vi "DMA Odometry Calculate.vi"(10 "Reset?":bool, 11 "Encoder Factor":dbl=1.0) -> (2 "Data Lost?":bool, 3 "Pose":T1)   [LabVIEW 2019]
uses:
  <vilib>/Rock Robotics/WPI/ThirdParty/WPILib Extensions/Geometry/Typedef/Pose2d.ctl
  <vilib>/Rock Robotics/WPI/ThirdParty/WPILib Extensions/Geometry/Typedef/Translation2d.ctl
  <vilib>/Rock Robotics/WPI/ThirdParty/WPILib Extensions/Geometry/Typedef/Rotation2d.ctl
  1db27cf9-0598-4eea-a655-fd467044f8ee.vi
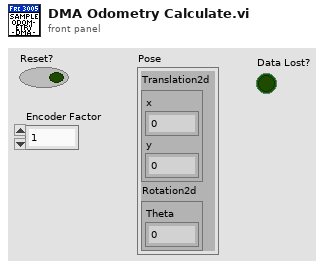
[diagram p1: front panel]
types:
  T1 = typedef "Pose2d.ctl" = cluster{"Translation2d":T2, "Rotation2d":T3}
  T2 = typedef "Translation2d.ctl" = cluster{"x":dbl, "y":dbl}
  T3 = typedef "Rotation2d.ctl" = cluster{"Theta":dbl}
  T4 = cluster{"Encoder R":i32, "Encoder L":i32, "Timestamp":u32}[]
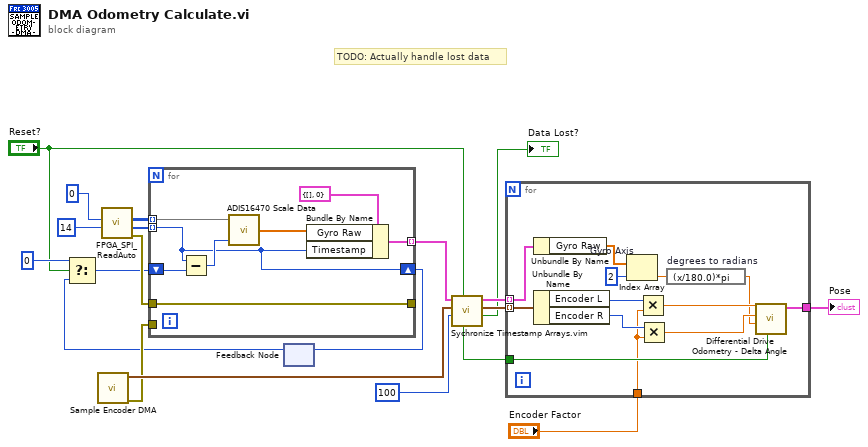
[diagram p0: block diagram]
diagram:
  # "TODO: Actually handle lost data"
  n1 = call "Sample Encoder DMA.vi"() -> ("error out"=w13:errorcluster, "Array"=w14:T4)  [unwired: 10 in]
  n2 = call <vilib>:"FPGA_SPI_ReadAuto.vi"("Bytes per Sample"=u32 14 ("Bytes Per Sample"), "Samples to Read"=u32 0) -> ("error out"=w12:errorcluster, "Timestamps"=w11:u32[], "Data"=w10:u8[][])  [unwired: 6 in, 1 out]
  n3 = feedback #1() -> (w4:u32)  [unwired: 1 in]
  n4 = Select(t=u32 0, s="Reset?", f=w4) -> (s? t:f=w3:u32)
  n5 = for {
    tunnel: w10 -> [w26] mode=indexing
    tunnel: w11 -> [w21] mode=indexing
    tunnel: w12 -> [w27]
    tunnel: [w27] -> _
    tunnel: w13 -> [_]
    tunnel: [w23] -> w15 mode=indexing
    shift-right: [w21] -> w5
    shift-left: w3 -> [w20]
    n6 = Subtract(x=w21, y=w20) -> (x-y=w22:u32)
    n7 = call "ADIS16470 Scale Data.vi"("TimeStamp"=w22, "Data In"=w26) -> ("Scaled Data Out"=w24:dbl[])  [unwired: 3 in]
    n8 = Bundle By Name(cluster=cluster{"Gyro Raw":dbl[], "Timestamp":u32} {"Gyro Raw"=[], "Timestamp"=0}, "Gyro Raw"=w24, "Timestamp"=w21) -> (w23:cluster{"Gyro Raw":dbl[], "Timestamp":u32})
  }
  n9 = feedback-in #1(w5) -> ()
  n10 = call "Sychronize Timestamp Arrays.vim"("Reset? (F)"="Reset?", "Timestamp Tolerance"=100, "Dataset 2"=w14, "Dataset 1"=w15) -> ("Data Lost?"=→"Data Lost?":bool, "Dataset 2 Out"=w17:T4, "Dataset 1 Out"=w16:cluster{"Gyro Raw":dbl[], "Timestamp":u32}[])  [unwired: 5 in]
  n11 = for {
    tunnel: w16 -> [w40] mode=indexing
    tunnel: w17 -> [w39] mode=indexing
    tunnel: "Reset?" -> [w35]
    tunnel: [w34] -> w18
    tunnel: "Encoder Factor" -> [w29]
    w37 = 2  # Gyro Axis
    n12 = Unbundle By Name(w40) -> ("Gyro Raw"=w38:dbl[])
    n13 = Unbundle By Name(w39) -> ("Encoder L"=w33:i32, "Encoder R"=w30:i32)
    n14 = Index Array(array=w38, index=w37) -> (element=w36:dbl)
    n15 = Multiply(x=w33, y=w29) -> (x*y=w32:dbl)
    n16 = Multiply(x=w30, y=w29) -> (x*y=w31:dbl)
    n17 = expression code="(x/180.0)*pi" "degrees to radians"(w36) -> (w28:dbl)
    n18 = call "Differential Drive Odometry - Delta Angle.vi"("Reset"=w35, "Delta Theta"=w28, "Right Distance"=w31, "Left Distance"=w32) -> ("Pose"=w34:T1)  [unwired: 7 in]
  }
  "Pose" <- w18
